vi "Modified Sync Filter k_j^n.vi"(9 "j":i32, 10 "m":i32, 11 "n":i32) -> (3 "k_j^(n)":dbl)   [LabVIEW 2021, in "Math.lvlib"]
uses:
  Math.lvlib
panel:
  # "see the License on the block diagram (Ctrl+E or Window:Show Block Diagram)"
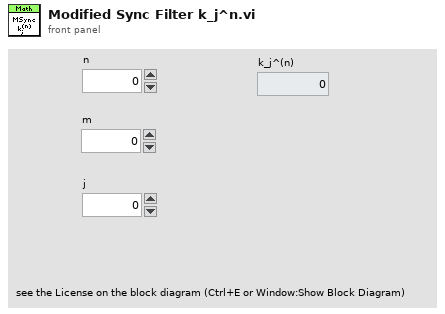
[diagram p1: front panel]
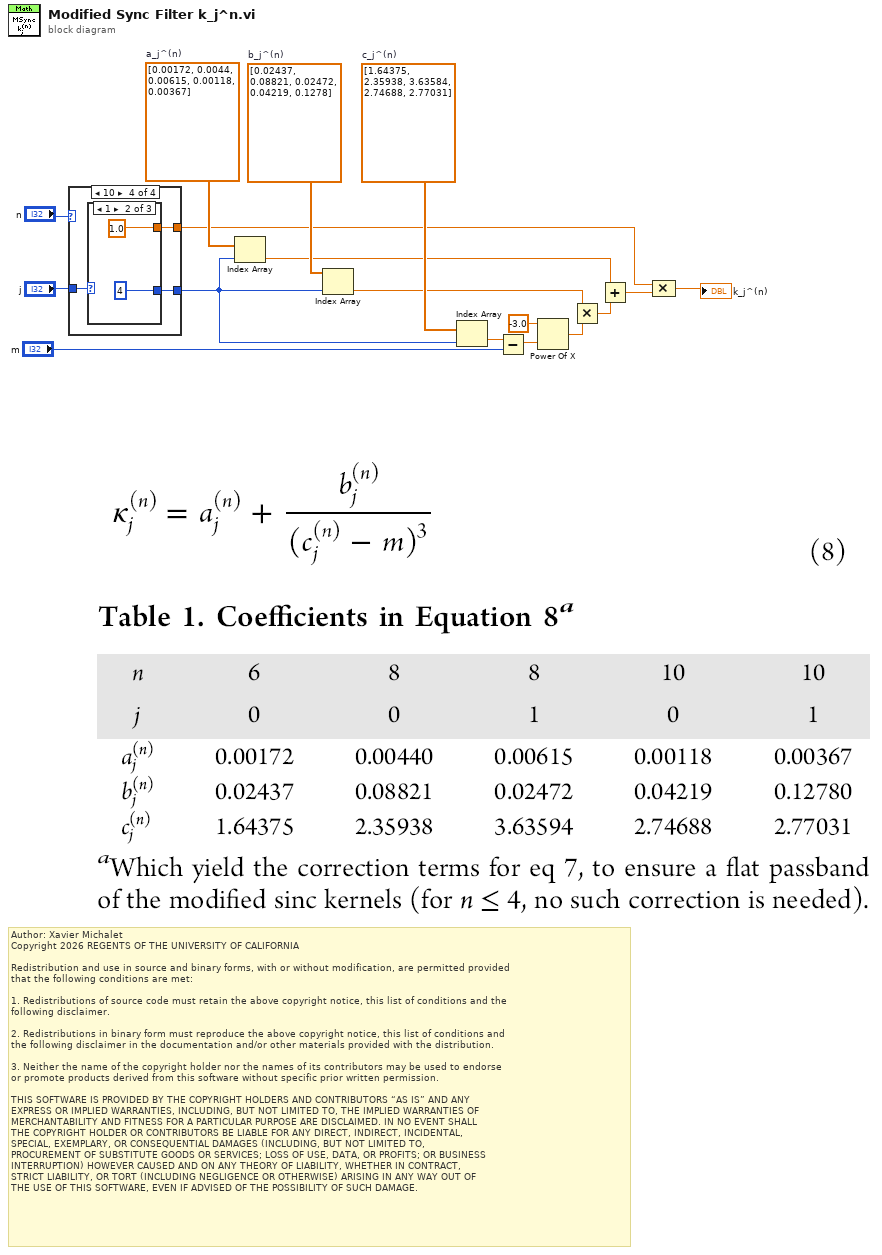
[diagram p0: block diagram]
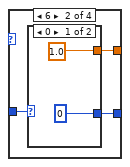
[diagram p3: hidden frame]
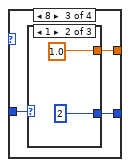
[diagram p5: hidden frame]
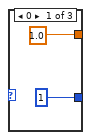
[diagram p6: hidden frame]
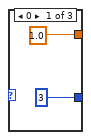
[diagram p8: hidden frame]
diagram:
  w15 = dbl[] [1.64375, 2.35938, 3.63584, 2.74688, 2.77031]  # c_j^(n)
  w16 = dbl[] [0.02437, 0.08821, 0.02472, 0.04219, 0.1278]  # b_j^(n)
  w17 = dbl[] [0.00172, 0.0044, 0.00615, 0.00118, 0.00367]  # a_j^(n)
  # "Author: Xavier Michalet\nCopyright 2026 REGENTS OF THE UNIVERSITY OF CALIFORNIA\n\nRedistribution and use in source and binary forms, with or without modification, are permitted provided\nthat the following conditions are met:\n\n1. Redistributions of source code must retain the above copyright notice, this list of conditions and the\nfollowing disclaimer.\n\n2. Redistributions in binary form must reproduce the above copyright notice, this list of conditions and\nthe following disclaimer in the documentation and/or other materials provided with the distribution.\n\n3. Neither the name of the copyright holder nor the names of its contributors may be used to endorse \nor promote products derived from this software without specific prior written permission.\n\nTHIS SOFTWARE IS PROVIDED BY THE COPYRIGHT HOLDERS AND CONTRIBUTORS “AS IS” AND ANY \nEXPRESS OR IMPLIED WARRANTIES, INCLUDING, BUT NOT LIMITED TO, THE IMPLIED WARRANTIES OF\nMERCHANTABILITY AND FITNESS FOR A PARTICULAR PURPOSE ARE DISCLAIMED. IN NO EVENT SHALL\nTHE COPYRIGHT HOLDER OR CONTRIBUTORS BE LIABLE FOR ANY DIRECT, INDIRECT, INCIDENTAL, \nSPECIAL, EXEMPLARY, OR CONSEQUENTIAL DAMAGES (INCLUDING, BUT NOT LIMITED TO, \nPROCUREMENT OF SUBSTITUTE GOODS OR SERVICES; LOSS OF USE, DATA, OR PROFITS; OR BUSINESS\nINTERRUPTION) HOWEVER CAUSED AND ON ANY THEORY OF LIABILITY, WHETHER IN CONTRACT, \nSTRICT LIABILITY, OR TORT (INCLUDING NEGLIGENCE OR OTHERWISE) ARISING IN ANY WAY OUT OF\nTHE USE OF THIS SOFTWARE, EVEN IF ADVISED OF THE POSSIBILITY OF SUCH DAMAGE."
  n1 = case shown="10" "n" {
    tunnel: [_ w20 w25 w32] -> w12
    tunnel: [_ w19 w24 w31] -> w2
    tunnel: "j" -> [_ w18 w23 w30]
    frame 0, Default {
    }
    frame 6 {
      n2 = case shown="0" w18 {
        tunnel: [0 ("index") _] -> w20
        tunnel: [1.0 ("element") _] -> w19
        frame 0 {
        }
        frame 1, Default {
        }
      }
    }
    frame 8 {
      n3 = case shown="1" w23 {
        tunnel: [1 ("index") 2 ("index") _] -> w25
        tunnel: [1.0 ("element") 1.0 ("element") _] -> w24
        frame 0 {
        }
        frame 1 {
        }
        frame 2, Default {
        }
      }
    }
    frame 10 {
      n4 = case shown="1" w30 {
        tunnel: [3 ("index") 4 ("index") _] -> w32
        tunnel: [1.0 ("element") 1.0 ("element") _] -> w31
        frame 0 {
        }
        frame 1 {
        }
        frame 2, Default {
        }
      }
    }
  }
  n5 = Index Array(array=w17, index=w12) -> (element=w6:dbl)
  n6 = Index Array(array=w16, index=w12) -> (element=w8:dbl)
  n7 = Index Array(array=w15, index=w12) -> (element=w11:dbl)
  n8 = Subtract(x=w11, y="m") -> (x-y=w10:dbl)
  n9 = Power Of X(1:w10, 2:-3.0 ("y")) -> (0:w7:dbl)
  n10 = Multiply(x=w8, y=w7) -> (x*y=w5:dbl)
  n11 = Add(x=w6, y=w5) -> (x+y=w13:dbl)
  n12 = Compound Arithmetic op=MULTIPLY(w2, w13) -> (→"k_j^(n)":dbl)
